vi "LoadModel.vi"(8 "error in (no error)":errorcluster, 10 "Actor In":refnum<class "Actor.lvclass">, 11 "GRMActor in":refnum<class "Controller Template.lvclass">) -> (0 "error out":errorcluster, 3 "GRMActor out":refnum<class "Controller Template.lvclass">)   [LabVIEW 2020, in "Controller Template.lvlib" / "Controller Template.lvclass"]
uses:
  Controller Template.lvclass
  <vilib>/ActorFramework/Actor/Actor.lvclass
  Model/Hardware Abstraction Layer/Component/GenericActor/GenericActor/GenericController.lvclass
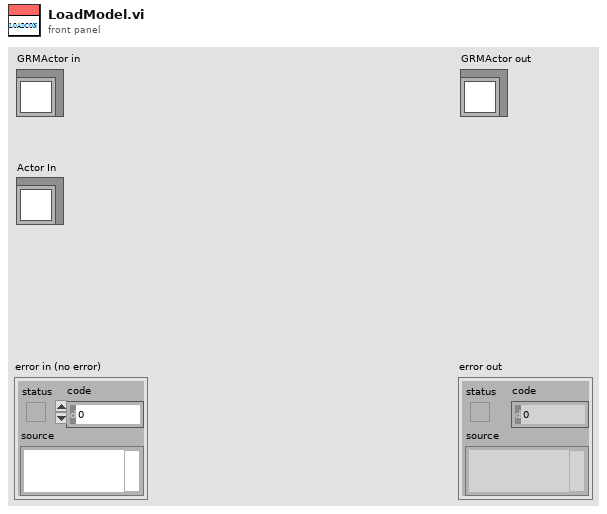
[diagram p1: front panel]
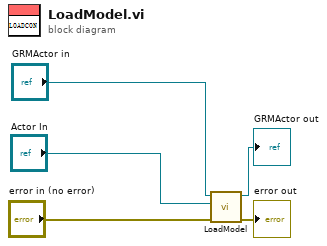
[diagram p0: block diagram]
diagram:
  n1 = call-parent "LoadModel.vi"("error in (no error)"="error in (no error)", "Actor In"="Actor In", "GRMActor in"="GRMActor in") -> ("error out"=→"error out":errorcluster, "GRMActor out"=→"GRMActor out":refnum<class "Controller Template.lvclass">)  [unwired: 7 in]
